vi "Create.vi"(7 "FIFO Options":T1, 8 "error in (no error)":errorcluster, 11 "fifo/queue depths (10)":u32=10) -> (0 "error out":errorcluster, 3 "Logging Interface out":refnum<class "Logging Interface.lvclass">)   [LabVIEW 2017, in "DSF Core.lvlib" / "Logging Interface.lvclass"]
uses:
  Logging Interface.lvclass
  C:/Git/DSF/Core/Classes/Interface/Interface.lvclass
  Typedefs/DSF FIFO Options.ctl
  Interface.lvclass
  Framework/Framework.lvclass
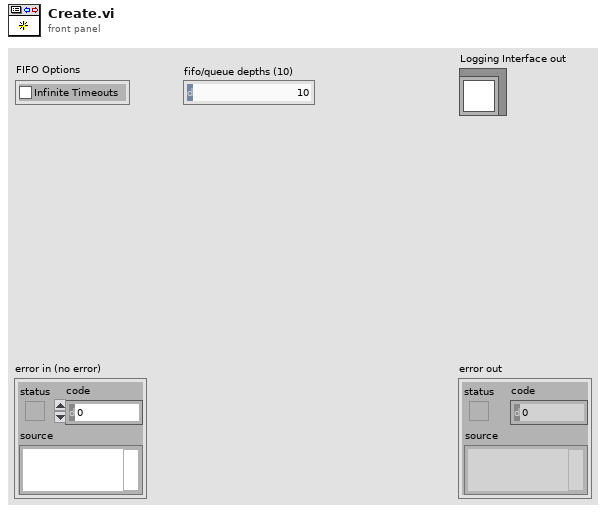
[diagram p1: front panel]
types:
  T1 = typedef "DSF Core.lvlib/Framework.lvclass/DSF FIFO Options.ctl" = cluster{"Infinite Timeouts":bool}
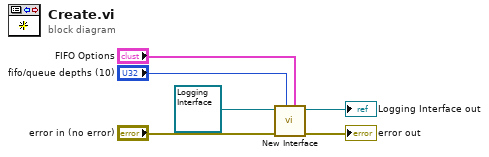
[diagram p0: block diagram]
diagram:
  n1 = call "New Interface.vi"("FIFO Options"="FIFO Options", "fifo/queue depths (10)"="fifo/queue depths (10)", "error in (no error)"="error in (no error)", "Interface type"=refnum<class "Logging Interface.lvclass"> refnum ("Logging Interface in")) -> ("error out"=→"error out":errorcluster, "Interface"=→"Logging Interface out":refnum<class "Logging Interface.lvclass">)  [unwired: 6 in]
